vi "FTW-JSON-LexicalScan-Pair.vi"(0 "JSON String":T1, 11 "error in":errorcluster) -> (4 "JSON String Out":T1, 6 "Name":string, 8 "Container":variant, 15 "error out":errorcluster)   [LabVIEW 2015]
uses:
  FTW-JSON-LexicalScan.ctl
panel:
  # "Inputs"
  # "Outputs"
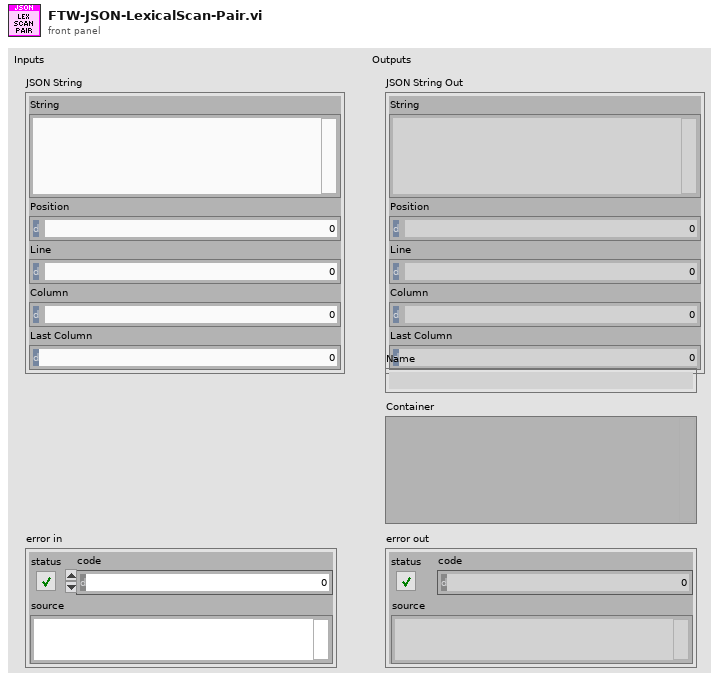
[diagram p1: front panel]
types:
  T1 = typedef "FTW-JSON-LexicalScan.ctl" = cluster{"String":string, "Position":i32, "Line":i32, "Column":i32, "Last Column":i32}
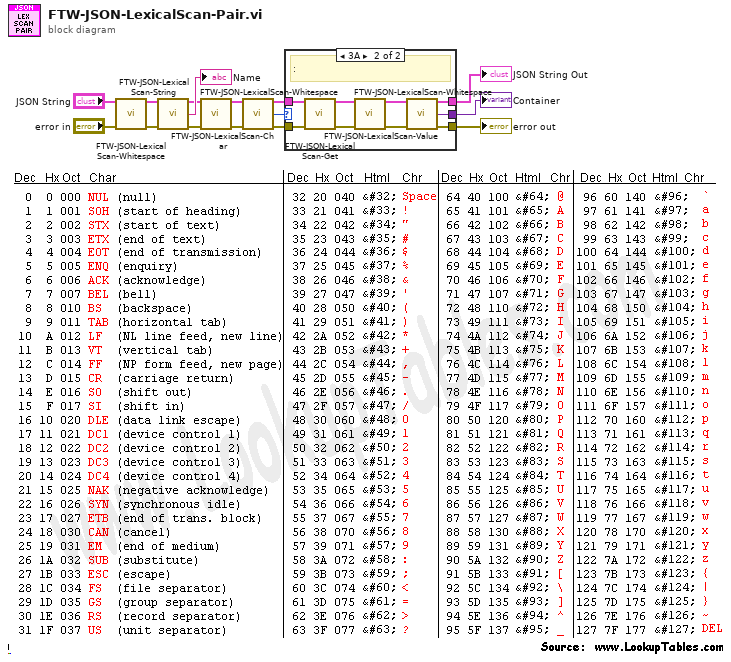
[diagram p0: block diagram]
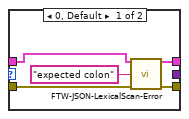
[diagram p2: hidden frame]
diagram:
  n1 = call "FTW-JSON-LexicalScan-Whitespace.vi"("JSON String"="JSON String", "error in"="error in") -> ("JSON String Out"=w11:T1, "error out"=w14:errorcluster)  [unwired: 12 in]
  n2 = call "FTW-JSON-LexicalScan-String.vi"("JSON String"=w11, "error in"=w14) -> ("JSON String Out"=w8:T1, "String"=→"Name":string, "error out"=w12:errorcluster)  [unwired: 11 in]
  n3 = call "FTW-JSON-LexicalScan-Whitespace.vi"("JSON String"=w8, "error in"=w12) -> ("JSON String Out"=w6:T1, "error out"=w9:errorcluster)  [unwired: 12 in]
  n4 = call "FTW-JSON-LexicalScan-Char.vi"("JSON String"=w6, "error in"=w9) -> ("JSON String Out"=w4:T1, "Char"=w2:u8, "error out"=w7:errorcluster)  [unwired: 11 in]
  n5 = case shown="3A" w2 {
    tunnel: w7 -> [w20 w29]
    tunnel: [w19 w24] -> w5
    tunnel: w4 -> [w18 w26]
    tunnel: [w17 w22] -> w3
    tunnel: [_ w21] -> w1
    frame 0, Default {
      n6 = call "FTW-JSON-LexicalScan-Error.vi"("JSON String"=w18, "Error String"="expected colon", "error in"=w20) -> ("JSON String Out"=w17:T1, "error out"=w19:errorcluster)  [unwired: 11 in]
    }
    frame 58 {
      # ":"
      n7 = call "FTW-JSON-LexicalScan-Get.vi"("JSON String"=w26, "error in"=w29) -> ("JSON String Out"=w25:T1, "error out"=w27:errorcluster)  [unwired: 11 in, 1 out]
      n8 = call "FTW-JSON-LexicalScan-Whitespace.vi"("JSON String"=w25, "error in"=w27) -> ("JSON String Out"=w23:T1, "error out"=w28:errorcluster)  [unwired: 12 in]
      n9 = call "FTW-JSON-LexicalScan-Value.vi"("JSON String"=w23, "error in"=w28) -> ("JSON String Out"=w22:T1, "Container"=w21:variant, "error out"=w24:errorcluster)  [unwired: 11 in]
    }
  }
  "Container" <- w1
  "error out" <- w5
  "JSON String Out" <- w3
